vi "X1.vi"(0 "denge degeri":dbl, 5 "Ýterasyon Denge":dbl, 7 "Xk":dbl, 9 "X(k-1)":dbl=0.1, 11 "output x 1":dbl) -> (4 "Output Xk":dbl, 6 "output x 2":dbl, 14 "cycle":bool, 15 "error":bool)   [LabVIEW 2014]
uses:
  Sub_VI/show_sensitivity.vi
  DB_Global_4_kart-Test.vi
  Global_input_values.vi
panel:
  out "cycle 2":bool
  in  "GPIB In":refnum<visa-resource-name>="GPIB0::8::INSTR"
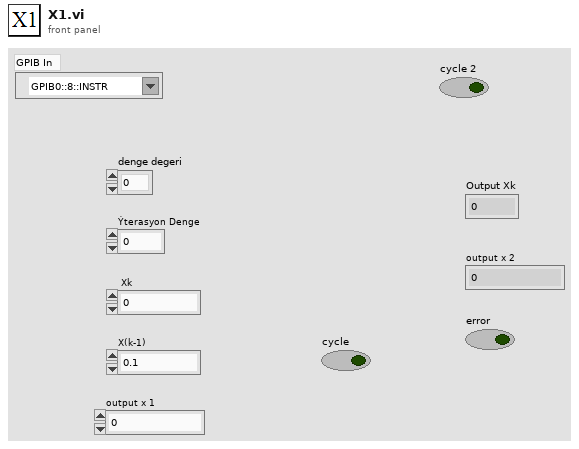
[diagram p1: front panel]
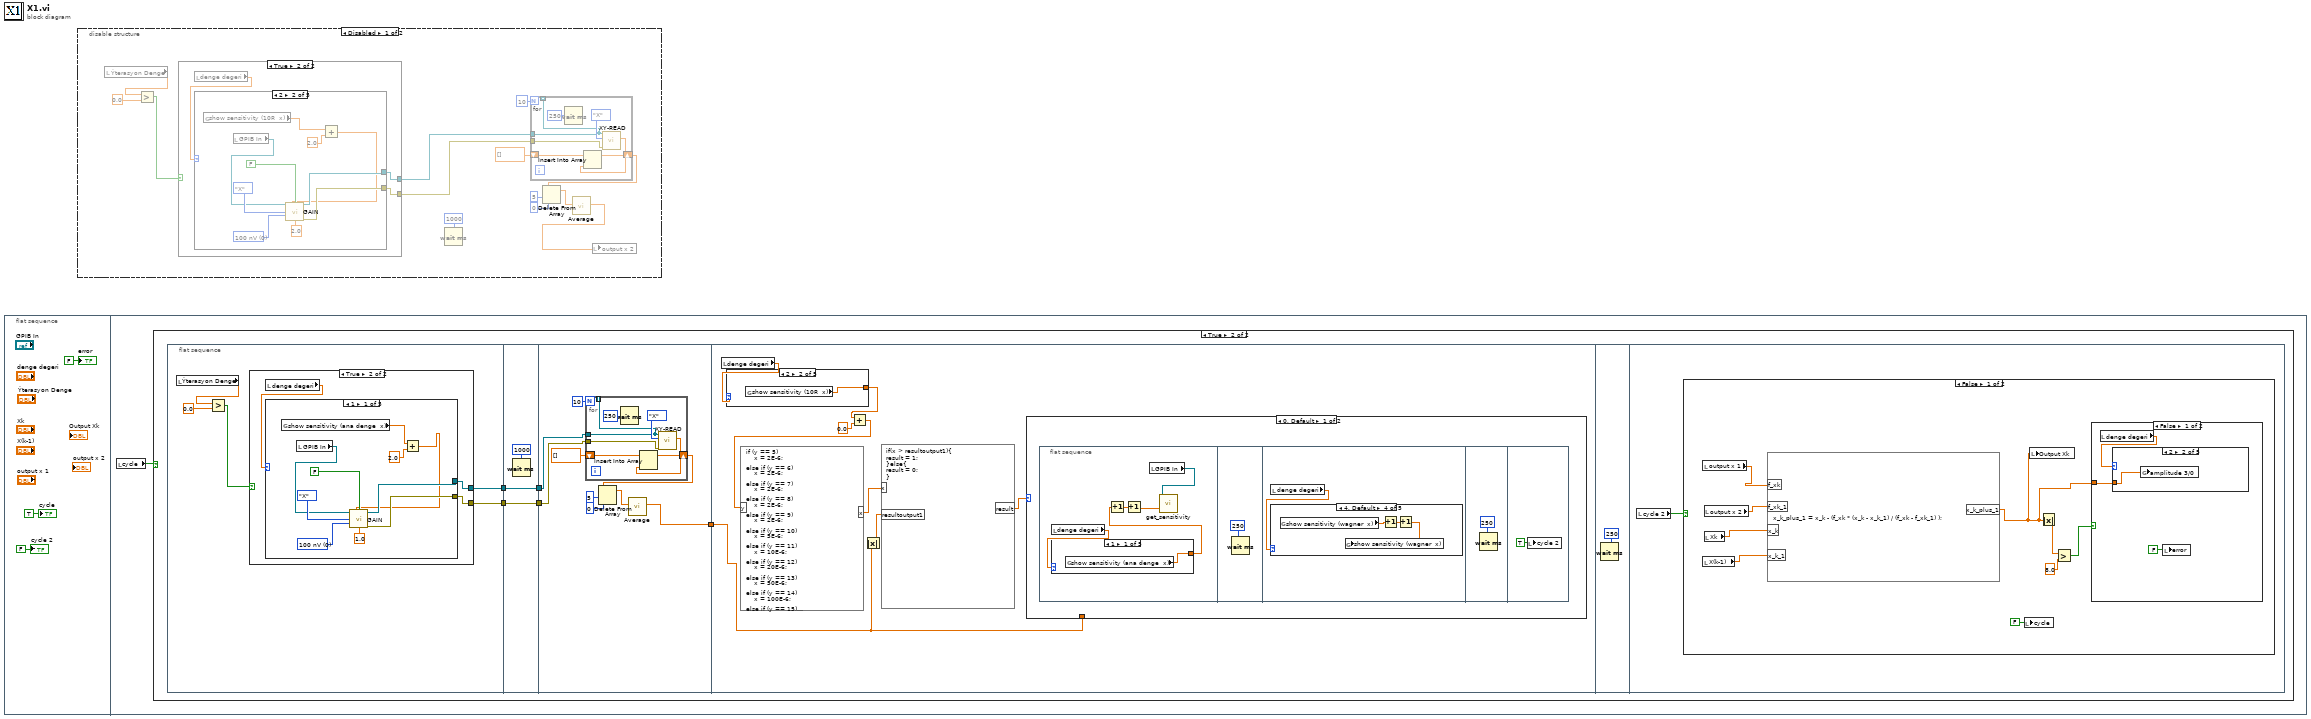
[diagram p0: block diagram]
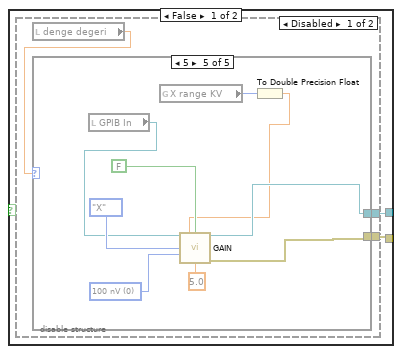
[diagram p2: hidden frame]
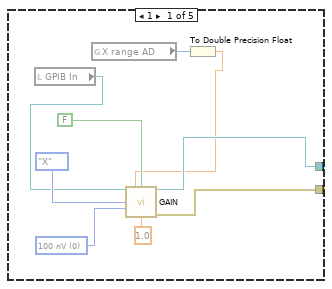
[diagram p3: hidden frame]
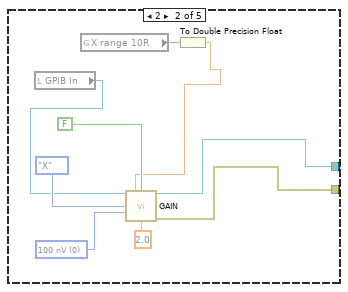
[diagram p4: hidden frame]
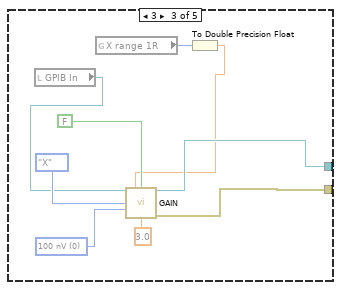
[diagram p5: hidden frame]
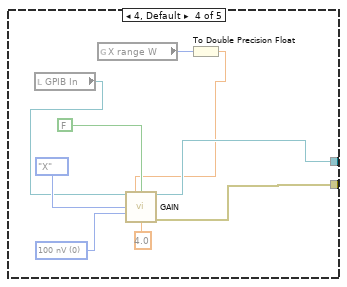
[diagram p6: hidden frame]
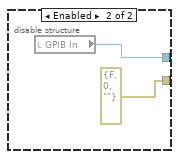
[diagram p7: hidden frame]
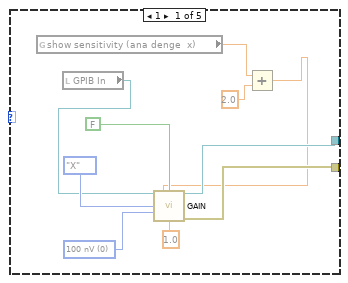
[diagram p8: hidden frame]
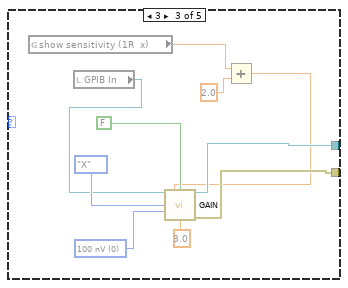
[diagram p9: hidden frame]
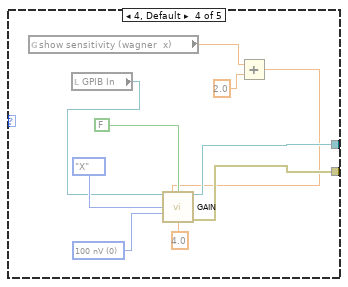
[diagram p10: hidden frame]
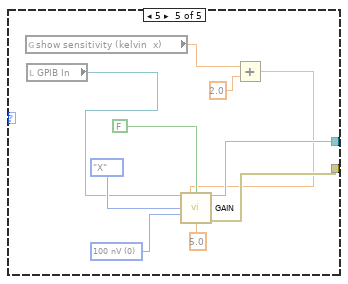
[diagram p11: hidden frame]
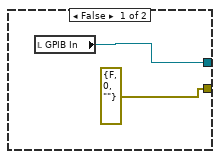
[diagram p14: hidden frame]
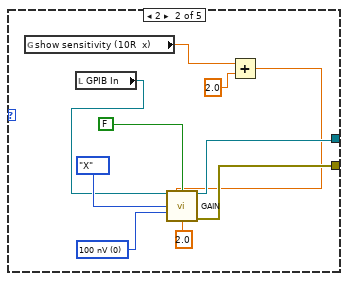
[diagram p15: hidden frame]
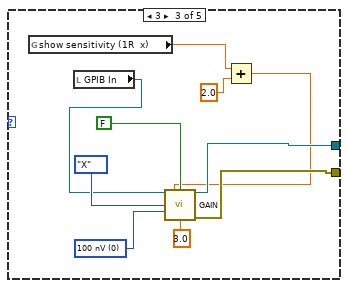
[diagram p16: hidden frame]
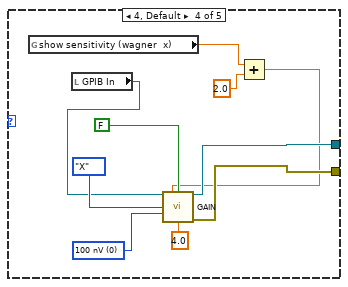
[diagram p17: hidden frame]
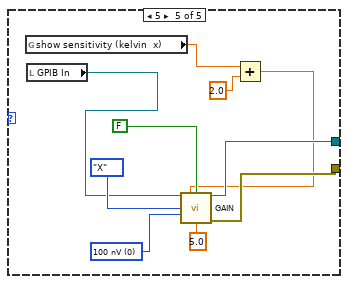
[diagram p18: hidden frame]
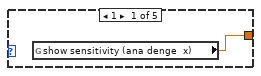
[diagram p19: hidden frame]
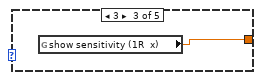
[diagram p20: hidden frame]
diagram:
  n1 = flat-sequence {
    frame #0 {
      "error" <- FALSE ("error")
      "cycle" <- TRUE ("error")
      "cycle 2" <- FALSE ("cycle 2")
    }
    frame #1 {
      n2 = local read "cycle"() -> (w4:bool)
      n3 = case shown="True" w4 {
        frame False {
        }
        frame True {
          n4 = flat-sequence {
            tunnel: [w11] -> w8
            tunnel: [w10] -> w6
            tunnel: [w71] -> w9
            tunnel: w8 -> [w71]
            tunnel: [w70] -> w7
            tunnel: w6 -> [w70]
            tunnel: w9 -> [w75]
            tunnel: w7 -> [w74]
            tunnel: [w73] -> w5
            tunnel: w5 -> [w90]
            frame #0 {
              n5 = local read "Ýterasyon Denge"() -> (w12:dbl)
              n6 = Greater?(x=w12, y=0.0) -> (0:w13:bool)
              n7 = case shown="True" w13 {
                tunnel: [w15 w18] -> w11
                tunnel: [errorcluster {"status"=FALSE, "code"=0, "source"=""} ("error out") w17] -> w10
                frame False {
                  n8 = local read "GPIB In"() -> (w15:refnum<visa-resource-name>)
                }
                frame True {
                  n9 = local read "denge degeri"() -> (w19:dbl)
                  n10 = case shown="1" w19 {
                    tunnel: [w24 w34 w44 w54 w65] -> w18
                    tunnel: [w23 w33 w43 w53 w64] -> w17
                    frame 1 {
                      w26 = u16 0 items=["100 nV", "200 nV", "500 nV", "1 uV", "2 uV", "5 uV", "10 uV", "20 uV", "50 uV", "100 uV", "200 uV", "500 uV", "1 mV"] ("Min. Hassasiyet")
                      n11 = global read "show_sensitivity.vi" "show sensitivity (ana denge  x)"() -> (w21:dbl)
                      n12 = local read "GPIB In"() -> (w27:refnum<visa-resource-name>)
                      n13 = Add(x=w21, y=2.0) -> (x+y=w20:dbl)
                      n14 = call "GAIN.vi"("SR850 GPIB In"=w27, "Max. Hassasiyet"=w20, "Auto Gain (False)"=FALSE, "Enum"=enum16{"X", "Y"}."X", "Min. Hassasiyet"=w26, "choose"=1.0) -> ("SR850 GPIB Out"=w24:refnum<visa-resource-name>, "error out"=w23:errorcluster)  [unwired: 7 in, 1 out]
                    }
                    frame 2 {
                      w36 = u16 0 items=["100 nV", "200 nV", "500 nV", "1 uV", "2 uV", "5 uV", "10 uV", "20 uV", "50 uV", "100 uV", "200 uV", "500 uV", "1 mV"] ("Min. Hassasiyet")
                      n15 = global read "show_sensitivity.vi" "show sensitivity (10R  x)"() -> (w31:dbl)
                      n16 = local read "GPIB In"() -> (w37:refnum<visa-resource-name>)
                      n17 = Add(x=w31, y=2.0) -> (x+y=w30:dbl)
                      n18 = call "GAIN.vi"("SR850 GPIB In"=w37, "Max. Hassasiyet"=w30, "Auto Gain (False)"=FALSE, "Enum"=enum16{"X", "Y"}."X", "Min. Hassasiyet"=w36, "choose"=2.0) -> ("SR850 GPIB Out"=w34:refnum<visa-resource-name>, "error out"=w33:errorcluster)  [unwired: 7 in, 1 out]
                    }
                    frame 3 {
                      w46 = u16 0 items=["100 nV", "200 nV", "500 nV", "1 uV", "2 uV", "5 uV", "10 uV", "20 uV", "50 uV", "100 uV", "200 uV", "500 uV", "1 mV"] ("Min. Hassasiyet")
                      n19 = global read "show_sensitivity.vi" "show sensitivity (1R  x)"() -> (w41:dbl)
                      n20 = local read "GPIB In"() -> (w47:refnum<visa-resource-name>)
                      n21 = Add(x=w41, y=2.0) -> (x+y=w40:dbl)
                      n22 = call "GAIN.vi"("SR850 GPIB In"=w47, "Max. Hassasiyet"=w40, "Auto Gain (False)"=FALSE, "Enum"=enum16{"X", "Y"}."X", "Min. Hassasiyet"=w46, "choose"=3.0) -> ("SR850 GPIB Out"=w44:refnum<visa-resource-name>, "error out"=w43:errorcluster)  [unwired: 7 in, 1 out]
                    }
                    frame 4, Default {
                      w56 = u16 0 items=["100 nV", "200 nV", "500 nV", "1 uV", "2 uV", "5 uV", "10 uV", "20 uV", "50 uV", "100 uV", "200 uV", "500 uV", "1 mV"] ("Min. Hassasiyet")
                      n23 = global read "show_sensitivity.vi" "show sensitivity (wagner  x)"() -> (w51:dbl)
                      n24 = local read "GPIB In"() -> (w57:refnum<visa-resource-name>)
                      n25 = Add(x=w51, y=2.0) -> (x+y=w50:dbl)
                      n26 = call "GAIN.vi"("SR850 GPIB In"=w57, "Max. Hassasiyet"=w50, "Auto Gain (False)"=FALSE, "Enum"=enum16{"X", "Y"}."X", "Min. Hassasiyet"=w56, "choose"=4.0) -> ("SR850 GPIB Out"=w54:refnum<visa-resource-name>, "error out"=w53:errorcluster)  [unwired: 7 in, 1 out]
                    }
                    frame 5 {
                      w67 = u16 0 items=["100 nV", "200 nV", "500 nV", "1 uV", "2 uV", "5 uV", "10 uV", "20 uV", "50 uV", "100 uV", "200 uV", "500 uV", "1 mV"] ("Min. Hassasiyet")
                      n27 = global read "show_sensitivity.vi" "show sensitivity (kelvin  x)"() -> (w61:dbl)
                      n28 = local read "GPIB In"() -> (w63:refnum<visa-resource-name>)
                      n29 = Add(x=w61, y=2.0) -> (x+y=w60:dbl)
                      n30 = call "GAIN.vi"("SR850 GPIB In"=w63, "Max. Hassasiyet"=w60, "Auto Gain (False)"=FALSE, "Enum"=enum16{"X", "Y"}."X", "Min. Hassasiyet"=w67, "choose"=5.0) -> ("SR850 GPIB Out"=w65:refnum<visa-resource-name>, "error out"=w64:errorcluster)  [unwired: 7 in, 1 out]
                    }
                  }
                }
              }
            }
            frame #1 {
              n31 = Wait (ms)(milliseconds to wait=u32 1000) -> ()  [unwired: 1 out]
            }
            frame #2 {
              n32 = for {
                N: 10 -> [_]
                shift-right: [w85] -> w79
                shift-left: dbl[] [] -> [w86]
                tunnel: [w83] -> _ mode=indexing
                tunnel: w75 -> [w83]
                tunnel: w74 -> [w82]
                n33 = Wait (ms)(milliseconds to wait=u32 250) -> ()  [unwired: 1 out]
                n34 = call "XY-READ.vi"("Error IN"=w82, "X/Y ?"=enum16{"X", "Y"}."X" ("Enum"), "SR850 GPIB IN"=w83) -> ("SR850_Reading"=w87:dbl)  [unwired: 6 in, 2 out]
                n35 = Insert Into Array(array=w86, new element=w87) -> (w85:dbl[])  [unwired: 1 in]
              }
              n36 = Delete From Array(array=w79, length=5, index=0) -> (array with subset deleted=w78:dbl[])  [unwired: 1 out]
              n37 = call "Average.vi"("Array"=w78) -> ("Average"=w73:dbl)  [unwired: 9 in, 1 out]
            }
            frame #3 {
              n38 = local read "denge degeri"() -> (w95:dbl)
              n39 = case shown="2" w95 {
                tunnel: [w97 w98 w99 w100 w101] -> w96
                frame 1 {
                  n40 = global read "show_sensitivity.vi" "show sensitivity (ana denge  x)"() -> (w97:dbl)
                }
                frame 2 {
                  n41 = global read "show_sensitivity.vi" "show sensitivity (10R  x)"() -> (w98:dbl)
                }
                frame 3 {
                  n42 = global read "show_sensitivity.vi" "show sensitivity (1R  x)"() -> (w99:dbl)
                }
                frame 4, Default {
                  n43 = global read "show_sensitivity.vi" "show sensitivity (wagner  x)"() -> (w100:dbl)
                }
                frame 5 {
                  n44 = global read "show_sensitivity.vi" "show sensitivity (kelvin  x)"() -> (w101:dbl)
                }
              }
              n45 = Add(x=w96, y=0.0) -> (x+y=w92:dbl)
              n46 = formula code="if (y == 5) \n    x = 2E-6;\n\nelse if (y == 6) \n    x = 2E-6;\n\nelse if (y == 7) \n    x = 2E-6;\n\nelse if (y == 8) \n    x = 2E-6;\n\nelse if (y == 9) \n    x = 2E-6;\n\nelse if (y == 10) \n    x = 5E-6;\n\nelse if (y == 11) \n    x = 10E-6;\n\nelse if (y == 12) \n    x = 20E-6;\n\nelse if (y == 13) \n    x = 50E-6;\n\nelse if (y == 14) \n    x = 100E-6;\n\nelse if (y == 15) \n    x = 200E-6;\n\nelse if (y == 16) \n    x = 500E-6;\n\nelse if (y == 17) \n    x = 1E-3;\n\nelse if (y == 18) \n    x = 2E-3;\n\nelse if (y == 19) \n    x = 5E-3;\n\nelse if (y == 20) \n    x = 10E-3;\n\nelse if (y == 21) \n    x = 20E-3;\n\nelse if (y == 22) \n    x = 50E-3;\n\nelse if (y == 23) \n    x = 100E-3;\n\nelse if (y == 24) \n    x = 200E-3;\n\nelse if (y == 25) \n    x = 500E-3;\n\nelse if (y == 26) \n    x = 1;\n\nelse \n    x = 1;"("y"=w92) -> ("x"=w94:dbl)
              n47 = Absolute Value(x=w90) -> (abs(x)=w89:dbl)
              n48 = formula code="if(x > resultoutput1){\nresult = 1;\n}else{\nresult = 0;\n}"("x"=w94, "resultoutput1"=w89) -> ("result"=w91:dbl)
              n49 = case shown="0, Default" w91 {
                tunnel: w90 -> [_ w131]
                frame 0, Default {
                  n50 = flat-sequence {
                    frame #0 {
                      n51 = local read "denge degeri"() -> (w104:dbl)
                      n52 = case shown="1" w104 {
                        tunnel: [w107 w108 w109 w110 w111] -> w103
                        frame 1 {
                          n53 = global read "show_sensitivity.vi" "show sensitivity (ana denge  x)"() -> (w107:dbl)
                        }
                        frame 2 {
                          n54 = global read "show_sensitivity.vi" "show sensitivity (10R  x)"() -> (w108:dbl)
                        }
                        frame 3 {
                          n55 = global read "show_sensitivity.vi" "show sensitivity (1R  x)"() -> (w109:dbl)
                        }
                        frame 4, Default {
                          n56 = global read "show_sensitivity.vi" "show sensitivity (wagner  x)"() -> (w110:dbl)
                        }
                        frame 5 {
                          n57 = global read "show_sensitivity.vi" "show sensitivity (kelvin  x)"() -> (w111:dbl)
                        }
                      }
                      n58 = Increment(x=w103) -> (x+1=w102:dbl)
                      n59 = Increment(x=w102) -> (x+1=w105:dbl)
                      n60 = local read "GPIB In"() -> (w106:refnum<visa-resource-name>)
                      n61 = call "get_sensitivity.vi"("input 1"=w105, "SR850 GPIB In"=w106) -> ()  [unwired: 8 in, 2 out]
                    }
                    frame #1 {
                      n62 = Wait (ms)(milliseconds to wait=u32 250) -> ()  [unwired: 1 out]
                    }
                    frame #2 {
                      n63 = local read "denge degeri"() -> (w113:dbl)
                      n64 = case shown="4, Default" w113 {
                        frame 1 {
                          n65 = global read "show_sensitivity.vi" "show sensitivity (ana denge  x)"() -> (w116:dbl)
                          n66 = Increment(x=w116) -> (x+1=w115:dbl)
                          n67 = Increment(x=w115) -> (x+1=w114:dbl)
                          n68 = global write "show_sensitivity.vi" "show sensitivity (ana denge  x)"(w114) -> ()
                        }
                        frame 2 {
                          n69 = global read "show_sensitivity.vi" "show sensitivity (10R  x)"() -> (w119:dbl)
                          n70 = Increment(x=w119) -> (x+1=w118:dbl)
                          n71 = Increment(x=w118) -> (x+1=w117:dbl)
                          n72 = global write "show_sensitivity.vi" "show sensitivity (10R  x)"(w117) -> ()
                        }
                        frame 3 {
                          n73 = global read "show_sensitivity.vi" "show sensitivity (1R  x)"() -> (w122:dbl)
                          n74 = Increment(x=w122) -> (x+1=w121:dbl)
                          n75 = Increment(x=w121) -> (x+1=w120:dbl)
                          n76 = global write "show_sensitivity.vi" "show sensitivity (1R  x)"(w120) -> ()
                        }
                        frame 4, Default {
                          n77 = global read "show_sensitivity.vi" "show sensitivity (wagner  x)"() -> (w125:dbl)
                          n78 = Increment(x=w125) -> (x+1=w124:dbl)
                          n79 = Increment(x=w124) -> (x+1=w123:dbl)
                          n80 = global write "show_sensitivity.vi" "show sensitivity (wagner  x)"(w123) -> ()
                        }
                        frame 5 {
                          n81 = global read "show_sensitivity.vi" "show sensitivity (kelvin  x)"() -> (w128:dbl)
                          n82 = Increment(x=w128) -> (x+1=w127:dbl)
                          n83 = Increment(x=w127) -> (x+1=w126:dbl)
                          n84 = global write "show_sensitivity.vi" "show sensitivity (kelvin  x)"(w126) -> ()
                        }
                      }
                    }
                    frame #3 {
                      n85 = Wait (ms)(milliseconds to wait=u32 250) -> ()  [unwired: 1 out]
                    }
                    frame #4 {
                      n86 = local write "cycle 2"(TRUE ("cycle")) -> ()
                    }
                  }
                }
                frame 1 {
                  n87 = local write "output x 2"(w131) -> ()
                  n88 = local write "cycle 2"(FALSE ("cycle")) -> ()
                }
              }
            }
            frame #4 {
              n89 = Wait (ms)(milliseconds to wait=u32 250) -> ()  [unwired: 1 out]
            }
            frame #5 {
              n90 = local read "cycle 2"() -> (w134:bool)
              n91 = case shown="False" w134 {
                frame False {
                  n92 = local read "output x 1"() -> (w138:dbl)
                  n93 = local read "X(k-1)"() -> (w136:dbl)
                  n94 = local read "output x 2"() -> (w139:dbl)
                  n95 = local read "Xk"() -> (w137:dbl)
                  n96 = formula code="x_k_plus_1 = x_k - (f_xk * (x_k - x_k_1) / (f_xk - f_xk_1) );"("f_xk"=w138, "f_xk_1"=w139, "x_k"=w137, "x_k_1"=w136) -> ("x_k_plus_1"=w140:dbl)
                  n97 = local write "cycle"(FALSE ("error")) -> ()
                  n98 = local write "Output Xk"(w140) -> ()
                  n99 = Absolute Value(x=w140) -> (abs(x)=w141:dbl)
                  n100 = Greater?(x=w141, y=8.0 ("Wagner  X(k-1)")) -> (0:w143:bool)
                  n101 = case shown="False" w143 {
                    tunnel: w140 -> [w144 _]
                    frame False {
                      n102 = local read "denge degeri"() -> (w146:dbl)
                      n103 = case shown="2" w146 {
                        tunnel: w144 -> [w147 w148 w149 w150 w151]
                        frame 1 {
                          n104 = global write "DB_Global_4_kart-Test.vi" "amplitude 2/0"(w147) -> ()
                        }
                        frame 2 {
                          n105 = global write "DB_Global_4_kart-Test.vi" "amplitude 3/0"(w148) -> ()
                        }
                        frame 3 {
                          n106 = global write "DB_Global_4_kart-Test.vi" "amplitude 3/1"(w149) -> ()
                        }
                        frame 4, Default {
                          n107 = global write "DB_Global_4_kart-Test.vi" "amplitude 1/1"(w150) -> ()
                        }
                        frame 5 {
                          n108 = global write "DB_Global_4_kart-Test.vi" "amplitude 2/1"(w151) -> ()
                        }
                      }
                      n109 = local write "error"(FALSE ("error")) -> ()
                    }
                    frame True {
                      n110 = local write "error"(TRUE ("error")) -> ()
                    }
                  }
                }
                frame True {
                  n111 = local write "cycle"(TRUE ("error")) -> ()
                }
              }
            }
          }
        }
      }
    }
  }
  n112 = disable-structure shown="Disabled" {
    frame Disabled {
      n113 = local read "Ýterasyon Denge"() -> (w166:dbl)
      n114 = Greater?(x=w166, y=0.0) -> (0:w165:bool)
      n115 = case shown="True" w165 {
        tunnel: [w168 w220] -> w161
        tunnel: [w167 w219] -> w162
        frame False {
          n116 = disable-structure shown="Disabled" {
            disable-tunnel: [w170 w218] -> w168
            disable-tunnel: [w169 errorcluster {"status"=FALSE, "code"=0, "source"=""} ("error out")] -> w167
            frame Disabled {
              n117 = local read "denge degeri"() -> (w171:dbl)
              n118 = case shown="5" w171 {
                tunnel: [w174 w184 w193 w202 w211] -> w170
                tunnel: [w175 w183 w192 w201 w210] -> w169
                frame 1 {
                  w177 = u16 0 items=["100 nV", "200 nV", "500 nV", "1 uV", "2 uV", "5 uV", "10 uV", "20 uV", "50 uV", "100 uV", "200 uV", "500 uV", "1 mV"] ("Min. Hassasiyet")
                  n119 = local read "GPIB In"() -> (w178:refnum<visa-resource-name>)
                  n120 = global read "Global_input_values.vi" "X range AD"() -> (w173:u8)
                  n121 = To Double Precision Float(number=w173) -> (double precision float=w172:dbl)
                  n122 = call "GAIN.vi"("SR850 GPIB In"=w178, "Max. Hassasiyet"=w172, "Auto Gain (False)"=FALSE, "Enum"=enum16{"X", "Y"}."X", "Min. Hassasiyet"=w177, "choose"=1.0) -> ("SR850 GPIB Out"=w174:refnum<visa-resource-name>, "error out"=w175:errorcluster)  [unwired: 7 in, 1 out]
                }
                frame 2 {
                  w186 = u16 0 items=["100 nV", "200 nV", "500 nV", "1 uV", "2 uV", "5 uV", "10 uV", "20 uV", "50 uV", "100 uV", "200 uV", "500 uV", "1 mV"] ("Min. Hassasiyet")
                  n123 = local read "GPIB In"() -> (w187:refnum<visa-resource-name>)
                  n124 = global read "Global_input_values.vi" "X range 10R"() -> (w182:u8)
                  n125 = To Double Precision Float(number=w182) -> (double precision float=w181:dbl)
                  n126 = call "GAIN.vi"("SR850 GPIB In"=w187, "Max. Hassasiyet"=w181, "Auto Gain (False)"=FALSE, "Enum"=enum16{"X", "Y"}."X", "Min. Hassasiyet"=w186, "choose"=2.0) -> ("SR850 GPIB Out"=w184:refnum<visa-resource-name>, "error out"=w183:errorcluster)  [unwired: 7 in, 1 out]
                }
                frame 3 {
                  w195 = u16 0 items=["100 nV", "200 nV", "500 nV", "1 uV", "2 uV", "5 uV", "10 uV", "20 uV", "50 uV", "100 uV", "200 uV", "500 uV", "1 mV"] ("Min. Hassasiyet")
                  n127 = local read "GPIB In"() -> (w196:refnum<visa-resource-name>)
                  n128 = global read "Global_input_values.vi" "X range 1R"() -> (w191:u8)
                  n129 = To Double Precision Float(number=w191) -> (double precision float=w190:dbl)
                  n130 = call "GAIN.vi"("SR850 GPIB In"=w196, "Max. Hassasiyet"=w190, "Auto Gain (False)"=FALSE, "Enum"=enum16{"X", "Y"}."X", "Min. Hassasiyet"=w195, "choose"=3.0) -> ("SR850 GPIB Out"=w193:refnum<visa-resource-name>, "error out"=w192:errorcluster)  [unwired: 7 in, 1 out]
                }
                frame 4, Default {
                  w204 = u16 0 items=["100 nV", "200 nV", "500 nV", "1 uV", "2 uV", "5 uV", "10 uV", "20 uV", "50 uV", "100 uV", "200 uV", "500 uV", "1 mV"] ("Min. Hassasiyet")
                  n131 = local read "GPIB In"() -> (w205:refnum<visa-resource-name>)
                  n132 = global read "Global_input_values.vi" "X range W"() -> (w200:u8)
                  n133 = To Double Precision Float(number=w200) -> (double precision float=w199:dbl)
                  n134 = call "GAIN.vi"("SR850 GPIB In"=w205, "Max. Hassasiyet"=w199, "Auto Gain (False)"=FALSE, "Enum"=enum16{"X", "Y"}."X", "Min. Hassasiyet"=w204, "choose"=4.0) -> ("SR850 GPIB Out"=w202:refnum<visa-resource-name>, "error out"=w201:errorcluster)  [unwired: 7 in, 1 out]
                }
                frame 5 {
                  w213 = u16 0 items=["100 nV", "200 nV", "500 nV", "1 uV", "2 uV", "5 uV", "10 uV", "20 uV", "50 uV", "100 uV", "200 uV", "500 uV", "1 mV"] ("Min. Hassasiyet")
                  n135 = local read "GPIB In"() -> (w214:refnum<visa-resource-name>)
                  n136 = global read "Global_input_values.vi" "X range KV"() -> (w209:u8)
                  n137 = To Double Precision Float(number=w209) -> (double precision float=w208:dbl)
                  n138 = call "GAIN.vi"("SR850 GPIB In"=w214, "Max. Hassasiyet"=w208, "Auto Gain (False)"=FALSE, "Enum"=enum16{"X", "Y"}."X", "Min. Hassasiyet"=w213, "choose"=5.0) -> ("SR850 GPIB Out"=w211:refnum<visa-resource-name>, "error out"=w210:errorcluster)  [unwired: 7 in, 1 out]
                }
              }
            }
            frame Enabled {
              n139 = local read "GPIB In"() -> (w218:refnum<visa-resource-name>)
            }
          }
        }
        frame True {
          n140 = local read "denge degeri"() -> (w221:dbl)
          n141 = case shown="2" w221 {
            tunnel: [w226 w236 w246 w256 w267] -> w220
            tunnel: [w225 w235 w245 w255 w266] -> w219
            frame 1 {
              w228 = u16 0 items=["100 nV", "200 nV", "500 nV", "1 uV", "2 uV", "5 uV", "10 uV", "20 uV", "50 uV", "100 uV", "200 uV", "500 uV", "1 mV"] ("Min. Hassasiyet")
              n142 = global read "show_sensitivity.vi" "show sensitivity (ana denge  x)"() -> (w223:dbl)
              n143 = local read "GPIB In"() -> (w229:refnum<visa-resource-name>)
              n144 = Add(x=w223, y=2.0) -> (x+y=w222:dbl)
              n145 = call "GAIN.vi"("SR850 GPIB In"=w229, "Max. Hassasiyet"=w222, "Auto Gain (False)"=FALSE, "Enum"=enum16{"X", "Y"}."X", "Min. Hassasiyet"=w228, "choose"=1.0) -> ("SR850 GPIB Out"=w226:refnum<visa-resource-name>, "error out"=w225:errorcluster)  [unwired: 7 in, 1 out]
            }
            frame 2 {
              w238 = u16 0 items=["100 nV", "200 nV", "500 nV", "1 uV", "2 uV", "5 uV", "10 uV", "20 uV", "50 uV", "100 uV", "200 uV", "500 uV", "1 mV"] ("Min. Hassasiyet")
              n146 = global read "show_sensitivity.vi" "show sensitivity (10R  x)"() -> (w233:dbl)
              n147 = local read "GPIB In"() -> (w239:refnum<visa-resource-name>)
              n148 = Add(x=w233, y=2.0) -> (x+y=w232:dbl)
              n149 = call "GAIN.vi"("SR850 GPIB In"=w239, "Max. Hassasiyet"=w232, "Auto Gain (False)"=FALSE, "Enum"=enum16{"X", "Y"}."X", "Min. Hassasiyet"=w238, "choose"=2.0) -> ("SR850 GPIB Out"=w236:refnum<visa-resource-name>, "error out"=w235:errorcluster)  [unwired: 7 in, 1 out]
            }
            frame 3 {
              w248 = u16 0 items=["100 nV", "200 nV", "500 nV", "1 uV", "2 uV", "5 uV", "10 uV", "20 uV", "50 uV", "100 uV", "200 uV", "500 uV", "1 mV"] ("Min. Hassasiyet")
              n150 = global read "show_sensitivity.vi" "show sensitivity (1R  x)"() -> (w243:dbl)
              n151 = local read "GPIB In"() -> (w249:refnum<visa-resource-name>)
              n152 = Add(x=w243, y=2.0) -> (x+y=w242:dbl)
              n153 = call "GAIN.vi"("SR850 GPIB In"=w249, "Max. Hassasiyet"=w242, "Auto Gain (False)"=FALSE, "Enum"=enum16{"X", "Y"}."X", "Min. Hassasiyet"=w248, "choose"=3.0) -> ("SR850 GPIB Out"=w246:refnum<visa-resource-name>, "error out"=w245:errorcluster)  [unwired: 7 in, 1 out]
            }
            frame 4, Default {
              w258 = u16 0 items=["100 nV", "200 nV", "500 nV", "1 uV", "2 uV", "5 uV", "10 uV", "20 uV", "50 uV", "100 uV", "200 uV", "500 uV", "1 mV"] ("Min. Hassasiyet")
              n154 = global read "show_sensitivity.vi" "show sensitivity (wagner  x)"() -> (w253:dbl)
              n155 = local read "GPIB In"() -> (w259:refnum<visa-resource-name>)
              n156 = Add(x=w253, y=2.0) -> (x+y=w252:dbl)
              n157 = call "GAIN.vi"("SR850 GPIB In"=w259, "Max. Hassasiyet"=w252, "Auto Gain (False)"=FALSE, "Enum"=enum16{"X", "Y"}."X", "Min. Hassasiyet"=w258, "choose"=4.0) -> ("SR850 GPIB Out"=w256:refnum<visa-resource-name>, "error out"=w255:errorcluster)  [unwired: 7 in, 1 out]
            }
            frame 5 {
              w269 = u16 0 items=["100 nV", "200 nV", "500 nV", "1 uV", "2 uV", "5 uV", "10 uV", "20 uV", "50 uV", "100 uV", "200 uV", "500 uV", "1 mV"] ("Min. Hassasiyet")
              n158 = global read "show_sensitivity.vi" "show sensitivity (kelvin  x)"() -> (w263:dbl)
              n159 = local read "GPIB In"() -> (w265:refnum<visa-resource-name>)
              n160 = Add(x=w263, y=2.0) -> (x+y=w262:dbl)
              n161 = call "GAIN.vi"("SR850 GPIB In"=w265, "Max. Hassasiyet"=w262, "Auto Gain (False)"=FALSE, "Enum"=enum16{"X", "Y"}."X", "Min. Hassasiyet"=w269, "choose"=5.0) -> ("SR850 GPIB Out"=w267:refnum<visa-resource-name>, "error out"=w266:errorcluster)  [unwired: 7 in, 1 out]
            }
          }
        }
      }
      n162 = Wait (ms)(milliseconds to wait=u32 1000) -> ()  [unwired: 1 out]
      n163 = for {
        N: 10 -> [_]
        shift-right: [w275] -> w156
        shift-left: dbl[] [] -> [w276]
        tunnel: [w273] -> _ mode=indexing
        tunnel: w161 -> [w273]
        tunnel: w162 -> [w272]
        n164 = Wait (ms)(milliseconds to wait=u32 250) -> ()  [unwired: 1 out]
        n165 = call "XY-READ.vi"("Error IN"=w272, "X/Y ?"=enum16{"X", "Y"}."X" ("Enum"), "SR850 GPIB IN"=w273) -> ("SR850_Reading"=w277:dbl)  [unwired: 6 in, 2 out]
        n166 = Insert Into Array(array=w276, new element=w277) -> (w275:dbl[])  [unwired: 1 in]
      }
      n167 = Delete From Array(array=w156, length=5, index=0) -> (array with subset deleted=w157:dbl[])  [unwired: 1 out]
      n168 = call "Average.vi"("Array"=w157) -> ("Average"=w160:dbl)  [unwired: 9 in, 1 out]
      n169 = local write "output x 2"(w160) -> ()
    }
    frame Enabled {
    }
  }
